vi "Select Range.vi"(7 "Channel (0: Channel A)":u16(ring) items=["Channel A", "Channel B"], 8 "error in (no error)":errorcluster, 10 "Range (0: Gauge)":u16(ring) items=["Gauge", "Pseudo-absolute"], 11 "BH Druck PACE Series in":refnum<class "BH Druck PACE Series.lvclass">) -> (0 "error out":errorcluster, 3 "BH Druck PACE Series out":refnum<class "BH Druck PACE Series.lvclass">)   [LabVIEW 2022 SP3, in "BH Druck PACE Series.lvclass"]
uses:
  BH Druck PACE Series.lvclass
  BH Druck PACE Series.lvclass/BH Druck PACE Series.ctl
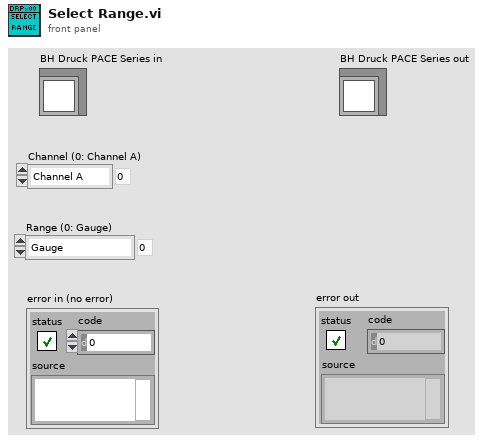
[diagram p1: front panel]
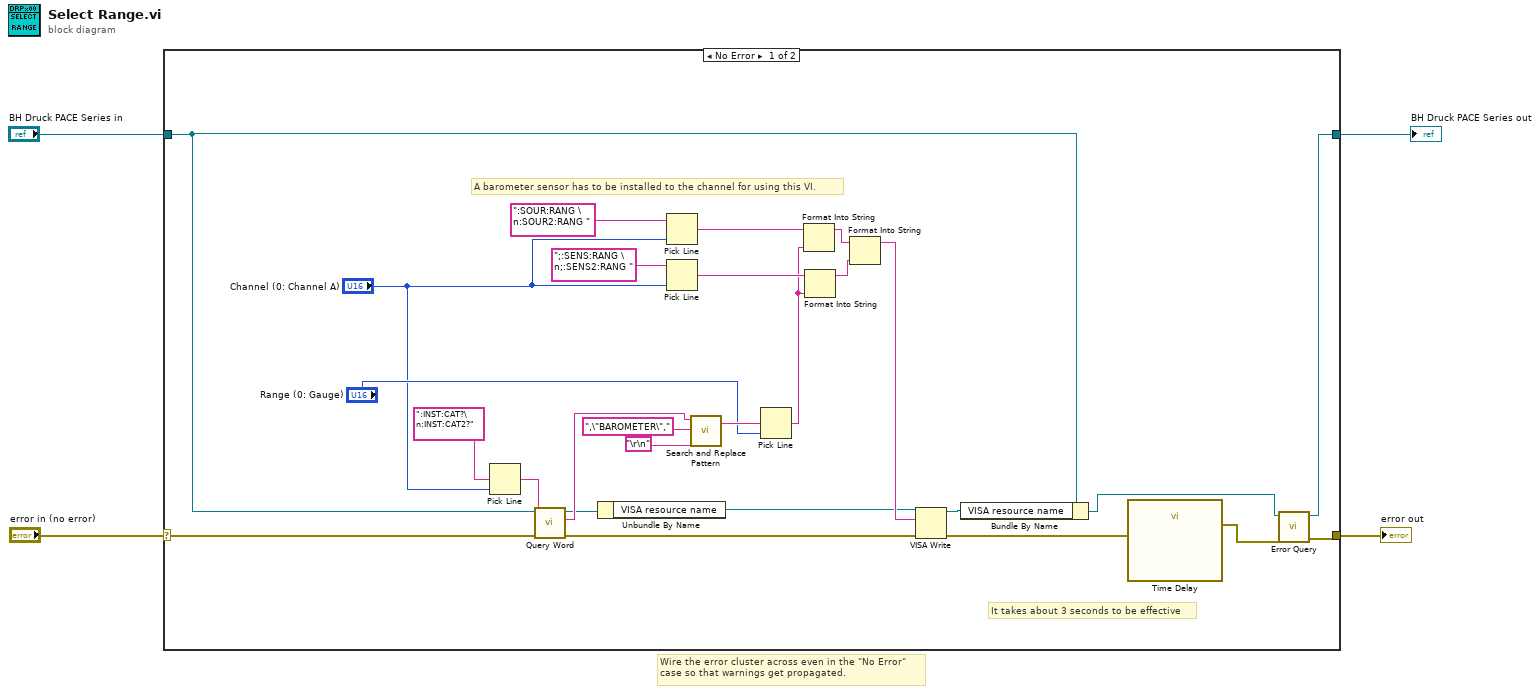
[diagram p0: block diagram]
diagram:
  # "Wire the error cluster across even in the \"No Error\"\ncase so that warnings get propagated."
  n1 = case shown="No Error" "error in (no error)" {
    selector: "error in (no error)" -> [w13 w33]
    tunnel: [w5 w33] -> w3
    tunnel: [w6 w32] -> w1
    tunnel: "BH Druck PACE Series in" -> [w10 w32]
    frame No Error {
      # "It takes about 3 seconds to be effective"
      # "A barometer sensor has to be installed to the channel for using this VI."
      n2 = Pick Line(multi-line string=":INST:CAT?\n:INST:CAT2?", line index="Channel (0: Channel A)") -> (output string=w19:string)  [unwired: 1 in]
      n3 = call-dynamic "Query Word.vi"("error in (no error)"=w13, "Query String"=w19, "BH Druck PACE Series in"=w10) -> ("error out"=w16:errorcluster, "String Result"=w17:string, "BH Druck PACE Series out"=w12:refnum<class "BH Druck PACE Series.lvclass">)  [unwired: 6 in]
      n4 = Unbundle By Name(w12) -> ("VISA resource name"=w11:refnum<visa-resource-name>)
      n5 = Pick Line(multi-line string=":SOUR:RANG \n:SOUR2:RANG ", line index="Channel (0: Channel A)") -> (output string=w25:string)  [unwired: 1 in]
      n6 = Pick Line(multi-line string=";:SENS:RANG \n;:SENS2:RANG ", line index="Channel (0: Channel A)") -> (output string=w24:string)  [unwired: 1 in]
      n7 = call <vilib>:"Search and Replace Pattern.vi"("string"=w17, "regular expression (\"\")"=",\"BAROMETER\"," ("regular expression (\"\")"), "replace string (\"\")"="\r\n" ("End of Line Constant")) -> ("result string"=w27:string)  [unwired: 2 in, 1 out]
      n8 = Pick Line(multi-line string=w27, line index="Range (0: Gauge)") -> (output string=w23:string)  [unwired: 1 in]
      n9 = Format Into String(initial string=w25, w23) -> (resulting string=w22:string)  [unwired: 2 in, 1 out]
      n10 = Format Into String(initial string=w24, w23) -> (resulting string=w21:string)  [unwired: 2 in, 1 out]
      n11 = Format Into String(initial string=w22, w21) -> (resulting string=w20:string)  [unwired: 2 in, 1 out]
      n12 = VISA Write(VISA resource name=w11, write buffer=w20, error in (no error)=w16) -> (VISA resource name out=w9:refnum<visa-resource-name>, error out=w14:errorcluster)  [unwired: 1 out]
      n13 = Bundle By Name(cluster=w10, "VISA resource name"=w9) -> (w7:refnum<class "BH Druck PACE Series.lvclass">)
      n14 = call "Time Delay"("error in (no error)"=w14) -> ("error out"=w8:errorcluster)  [unwired: 10 in]
      n15 = call-dynamic "Error Query.vi"("error in (no error)"=w8, "BH Druck PACE Series in"=w7) -> ("error out"=w5:errorcluster, "BH Druck PACE Series out"=w6:refnum<class "BH Druck PACE Series.lvclass">)  [unwired: 8 in]
    }
    frame Error {
    }
  }
  "error out" <- w3
  "BH Druck PACE Series out" <- w1
